vi "Read Array of Launch Instrument Addresses.vi"(8 "error in (no error)":errorcluster, 11 "Instrument Finder in":refnum<class "Instrument Finder.lvclass">) -> (0 "error out":errorcluster, 2 "Array of Launch Instrument Addresses":refnum<class "Message Enqueuer.lvclass">[](array[class]), 3 "Instrument Finder out":refnum<class "Instrument Finder.lvclass">)   [LabVIEW 2014, in "SetUp VIs.lvlib" / "Instrument Finder.lvclass"]
uses:
  Instrument Finder.lvclass
  <vilib>/ActorFramework/Message Enqueuer/Message Enqueuer.lvclass
  Instrument Finder.lvclass/Instrument Finder.ctl
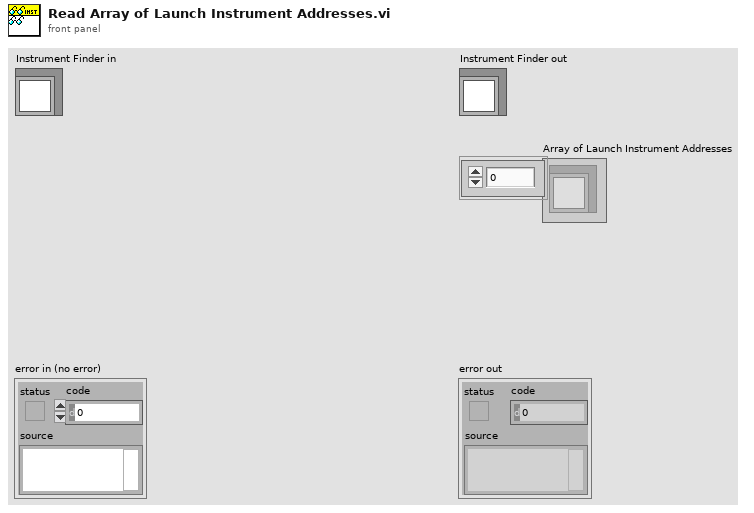
[diagram p1: front panel]
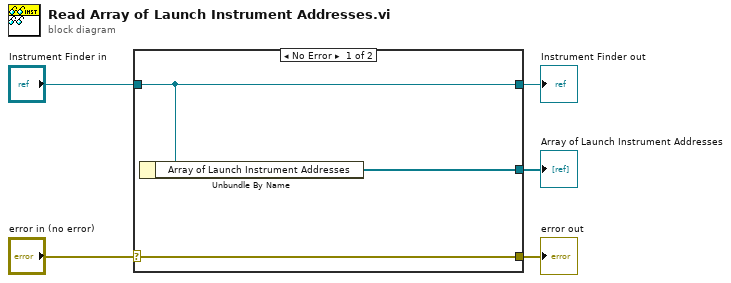
[diagram p0: block diagram]
diagram:
  n1 = case shown="No Error" "error in (no error)" {
    selector: "error in (no error)" -> [w8 w9]
    tunnel: [w8 w9] -> w4
    tunnel: [w7 w10] -> w2
    tunnel: "Instrument Finder in" -> [w7 w10]
    tunnel: [w6 _] -> w1
    frame No Error {
      n2 = Unbundle By Name(w7) -> ("Array of Launch Instrument Addresses"=w6:refnum<class "Message Enqueuer.lvclass">[])
    }
    frame Error {
    }
  }
  "error out" <- w4
  "Instrument Finder out" <- w2
  "Array of Launch Instrument Addresses" <- w1
